vi "SubVI_Train_SVM.vi"(0 "Rest Epochs":dbl[][](array[numeric]), 1 "Repeat training?":bool=TRUE, 5 "Go Epochs in":dbl[][](array[numeric]), 9 "Max Passes":i32=15, 11 "error in (no error)":errorcluster, 12 "Gamma":dbl[](array[numeric])=[1.0, 5.0, 10.0, 50.0, 100.0, 0.2, 0.5, 0.8], 13 "C":dbl[](array[numeric])=[0.1, 1.0, 10.0, 100.0, 1000.0], 14 "Optimizer\nMetric":string="F1") -> (3 "Go Epochs out":dbl[][](array[numeric]), 4 "Hyperparameters":T1, 6 "Best (Metric)":dbl, 10 "Optimum Window Size":i32, 15 "error out":errorcluster)   [LabVIEW 2020]
uses:
  <vilib>/Analysis/Matrix/Numeric/Conversions/Matrix To Array - RM.vi
  Global 1.vi
  <vilib>/gmath/NI_Gmath.lvlib
  <vilib>/Analysis/Matrix/NI_Matrix.lvlib
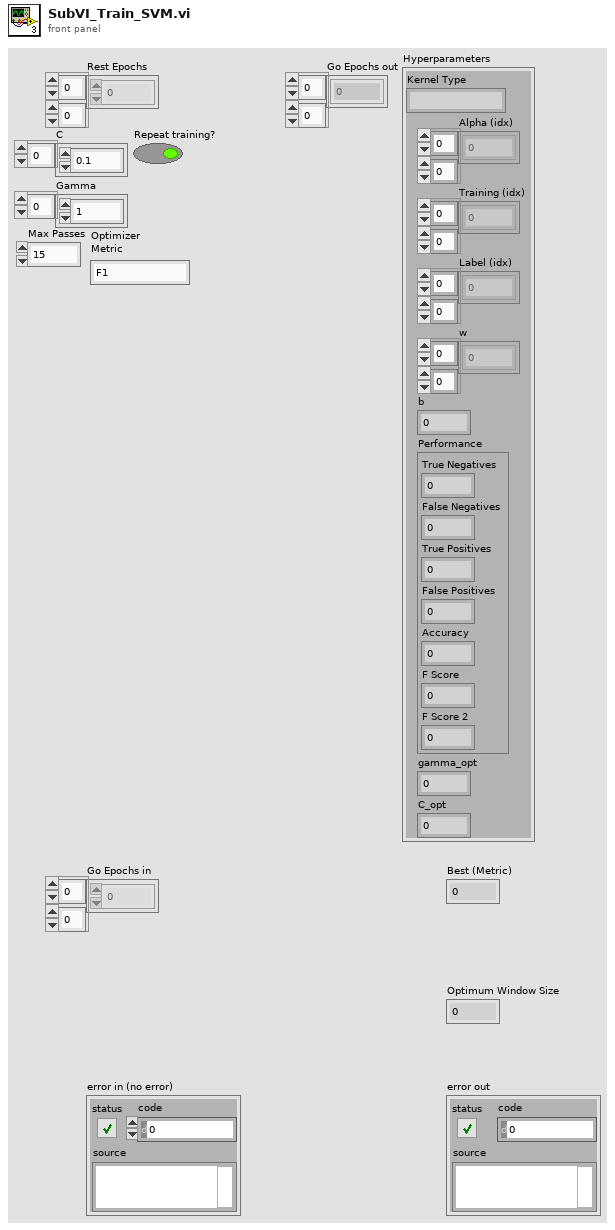
[diagram p1: front panel]
types:
  T1 = cluster{"Kernel Type":string, "Alpha (idx)":dbl[][], "Training (idx)":dbl[][], "Label (idx)":dbl[][], "w":dbl[][], "b":dbl, "Performance":cluster{"True Negatives":i32, "False Negatives":i32, "True Positives":i32, "False Positives":i32, "Accuracy":dbl, "F Score":dbl, "F Score 2":dbl}, "gamma_opt":dbl, "C_opt":dbl}
  T2 = typedef "NI_Matrix.lvlib/RealMatrix.ctl" = dbl[][]
  T3 = cluster{"True Negatives":i32, "False Negatives":i32, "True Positives":i32, "False Positives":i32, "Accuracy":dbl, "F1 Score":dbl, "Precision":dbl}
  T4 = cluster{"Kernel Type":string, "Alpha (idx)":dbl[][], "Training (idx)":dbl[][], "Label (idx)":dbl[][], "w":dbl[][], "b":dbl, "Performance":cluster{"True Negatives":i32, "False Negatives":i32, "True Positives":i32, "False Positives":i32, "Accuracy":dbl, "F1 Score":dbl, "Precision":dbl}, "gamma_opt":dbl, "C_opt":dbl}
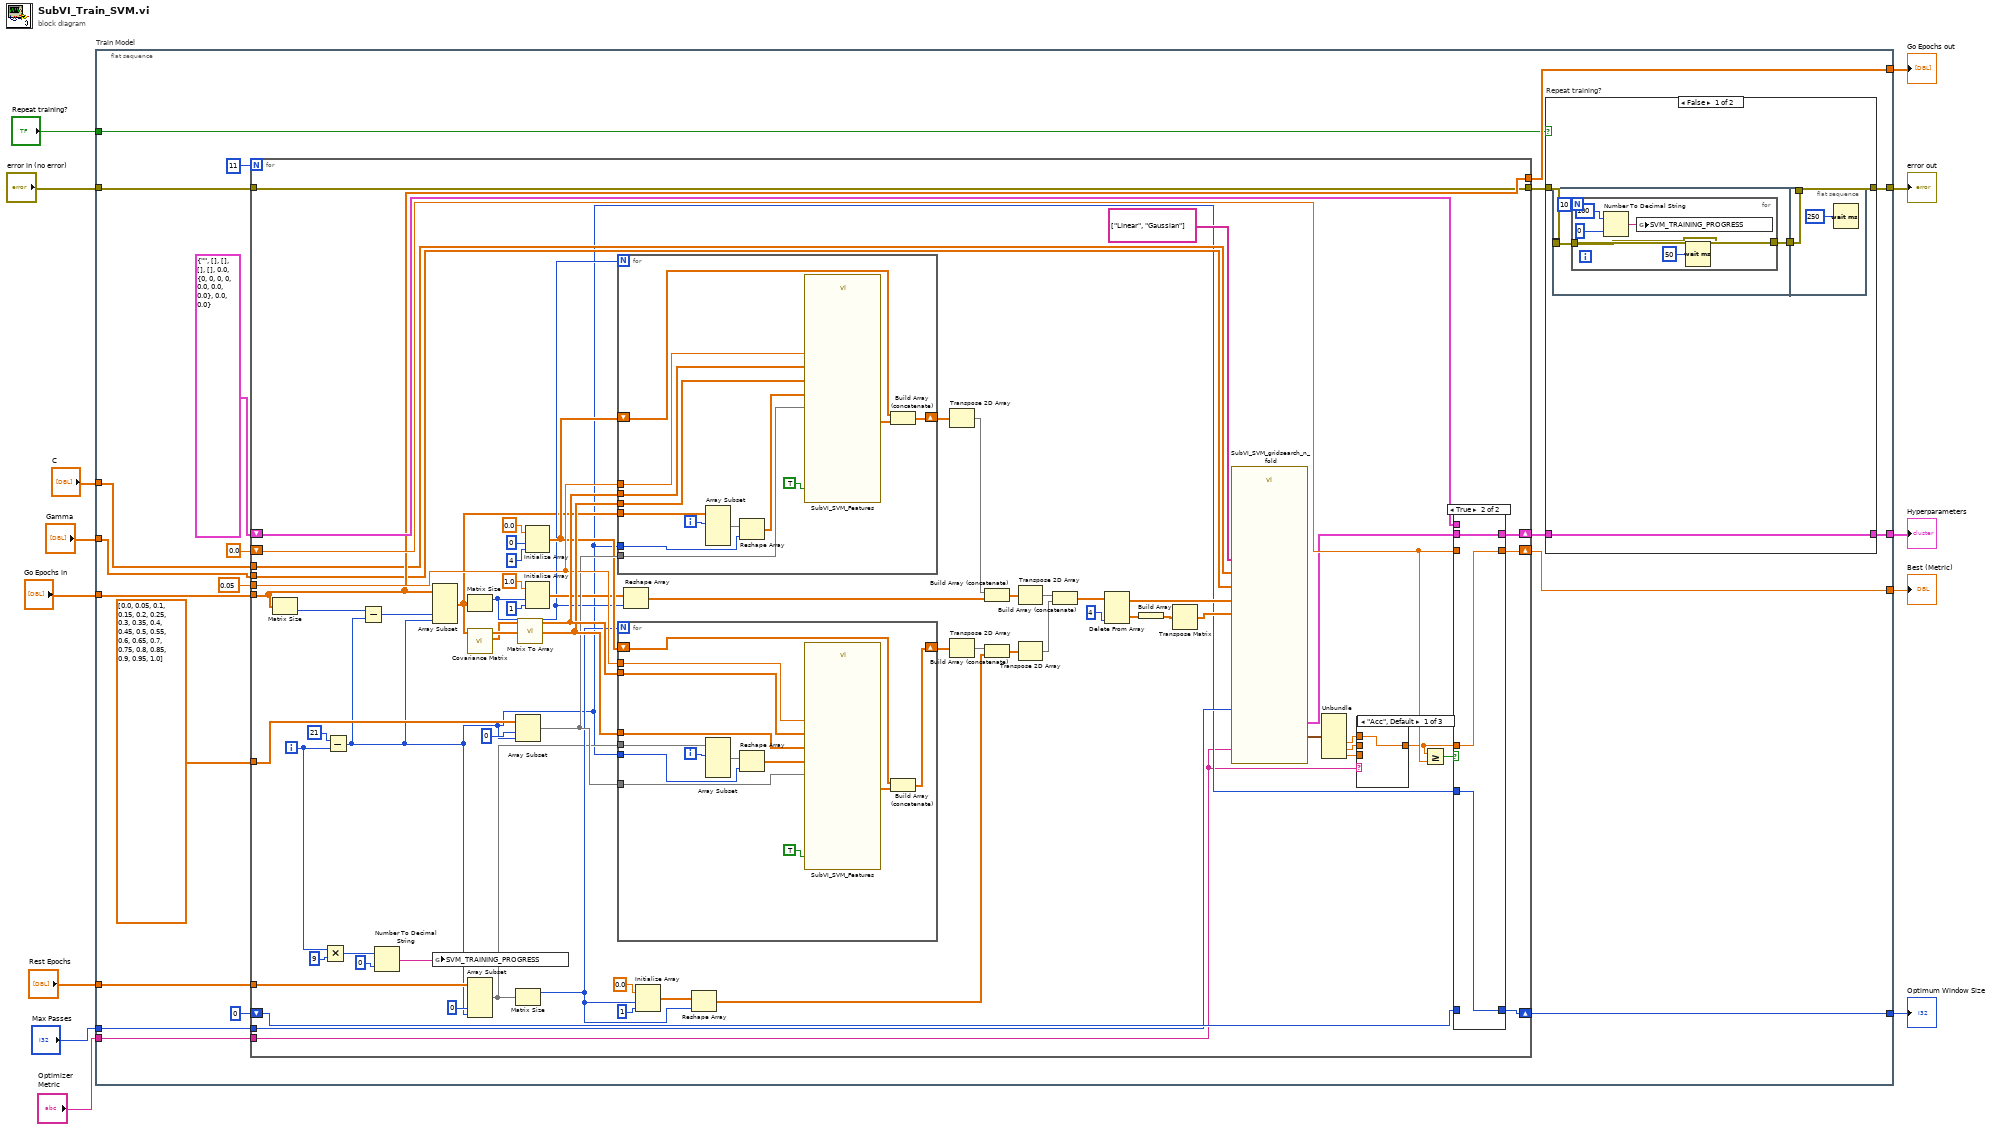
[diagram p0: block diagram]
diagram:
  n1 = flat-sequence "Train Model" {
    tunnel: "Go Epochs in" -> [w29]
    tunnel: "Rest Epochs" -> [w28]
    tunnel: [w27] -> w7
    tunnel: [w21] -> w2
    tunnel: [w26] -> w8
    tunnel: [w25] -> w9
    tunnel: [w15] -> w12
    tunnel: "error in (no error)" -> [w23]
    tunnel: "C" -> [w20]
    tunnel: "Gamma" -> [w19]
    tunnel: "Max Passes" -> [w18]
    tunnel: "Repeat training?" -> [w17]
    tunnel: "Optimizer\nMetric" -> [w14]
    frame #0 {
      n2 = for {
        N: 11 -> [_]
        tunnel: w29 -> [w71]
        tunnel: dbl[] [0.0, 0.05, 0.1, 0.15, 0.2, 0.25, 0.3, 0.35, 0.4, 0.45, 0.5, 0.55, 0.6, 0.65, 0.7, 0.75, 0.8, 0.85, 0.9, 0.95, 1.0] ("Sliding_window") -> [w117]
        tunnel: 0.05 ("dt") -> [w112]
        tunnel: w28 -> [w110]
        shift-right: [w75] -> w22
        shift-left: T1 {"Kernel Type"="", "Alpha (idx)"=[], "Training (idx)"=[], "Label (idx)"=[], "w"=[], "b"=0.0, "Performance"={"True Negatives"=0, "False Negatives"=0, "True Positives"=0, "False Positives"=0, "Accuracy"=0.0, "F Score"=0.0, "F Score 2"=0.0}, "gamma_opt"=0.0, "C_opt"=0.0} ("Hyperparameters") -> [w78]
        shift-right: [w73] -> w27
        shift-left: 0.0 -> [w74]
        shift-right: [w76] -> w25
        shift-left: 0 -> [w77]
        tunnel: [w71] -> w26
        tunnel: [w68] -> w16
        tunnel: w23 -> [w68]
        tunnel: w20 -> [w61]
        tunnel: w19 -> [w60]
        tunnel: w18 -> [w59]
        tunnel: w14 -> [w51]
        i -> [w63]
        n3 = Matrix Size(0:w71) -> (2:w69:i32)  [unwired: 1 out]
        n4 = Multiply(x=w63, y=9) -> (x*y=w64:i32)
        n5 = Subtract(x=21, y=w63) -> (x-y=w56:i32)
        n6 = Subtract(x=w69, y=w56) -> (x-y=w70:i32)
        n7 = Number To Decimal String(number=w64, width (-)=i16 0) -> (decimal integer string=w65:string)
        n8 = Array Subset(array=w71, index (col)=w70, length (col)=w56) -> (w87:dbl[][])  [unwired: 2 in]
        n9 = global write "Global 1.vi" "SVM_TRAINING_PROGRESS"(w65) -> ()
        n10 = Matrix Size(0:w87) -> (1:w90:i32)  [unwired: 1 out]
        n11 = call <vilib>:"Covariance Matrix.vi"("X"=w87) -> ("mean vector"=w114:dbl[], "covariance matrix V"=w118:T2)  [unwired: 9 in]
        n12 = Array Subset(array=w110, index (col)=0 ("index"), length (col)=w56) -> (w88:dbl[][])  [unwired: 2 in]
        n13 = Array Subset(array=w117, index=0, length=w56) -> (w109:dbl[])
        n14 = Matrix Size(0:w88) -> (1:w91:i32)  [unwired: 1 out]
        n15 = call-poly <vilib>:"Matrix To Array.vi"("Real Matrix"=w118) -> ("Real 2D Array"=w113:dbl[][])
        n16 = Initialize Array(0.0 ("element"), 0 ("dimension size"), 4 ("dimension size")) -> (w105:dbl[][])
        n17 = Initialize Array(1.0 ("element"), w90, 1 ("dimension size")) -> (w95:dbl[][])
        n18 = for {
          N: w90 -> [_]
          tunnel: w114 -> [w139]
          tunnel: w113 -> [w137]
          tunnel: w112 -> [w140]
          tunnel: w109 -> [w138]
          shift-right: [w135] -> w89
          shift-left: w105 -> [w136]
          tunnel: w87 -> [w133]
          tunnel: w56 -> [w131]
          i -> [w130]
          n19 = Array Subset(array=w133, index (row)=w130) -> (w132:dbl[][])  [unwired: 3 in]
          n20 = Reshape Array(w132, w131) -> (w129:dbl[])
          n21 = call "SubVI_SVM_Features.vi"("Sigma"=w137, "MU"=w139, "Scale?"=TRUE, "dt"=w140, "window_time"=w138, "Sliding_window"=w129) -> ("Features_array"=w134:dbl[])  [unwired: 1 in, 4 out]
          n22 = Build Array (concatenate)(w136, w134) -> (w135:dbl[][])
        }
        n23 = for {
          N: w91 -> [_]
          tunnel: w114 -> [w153]
          tunnel: w113 -> [w148]
          tunnel: w112 -> [w142]
          tunnel: w109 -> [w152]
          shift-right: [w149] -> w98
          shift-left: w105 -> [w151]
          tunnel: w88 -> [w147]
          tunnel: w56 -> [w143]
          i -> [w146]
          n24 = Array Subset(array=w147, index (row)=w146) -> (w145:dbl[][])  [unwired: 3 in]
          n25 = Reshape Array(w145, w143) -> (w144:dbl[])
          n26 = call "SubVI_SVM_Features.vi"("Sigma"=w148, "MU"=w153, "Scale?"=TRUE, "dt"=w142, "window_time"=w152, "Sliding_window"=w144) -> ("Features_array"=w150:dbl[])  [unwired: 1 in, 4 out]
          n27 = Build Array (concatenate)(w151, w150) -> (w149:dbl[][])
        }
        n28 = Reshape Array(w95, w90) -> (w94:dbl[])
        n29 = Initialize Array(0.0 ("element"), w91, 1 ("dimension size")) -> (w102:dbl[][])
        n30 = Reshape Array(w102, w91) -> (w101:dbl[])
        n31 = Transpose 2D Array(2D array=w89) -> (transposed array=w93:dbl[][])
        n32 = Transpose 2D Array(2D array=w98) -> (transposed array=w100:dbl[][])
        n33 = Build Array (concatenate)(w93, w94) -> (w92:dbl[][])
        n34 = Build Array (concatenate)(w100, w101) -> (w99:dbl[][])
        n35 = Transpose 2D Array(2D array=w92) -> (transposed array=w86:dbl[][])
        n36 = Transpose 2D Array(2D array=w99) -> (transposed array=w85:dbl[][])
        n37 = Build Array (concatenate)(w86, w85) -> (w84:dbl[][])
        n38 = Delete From Array(array=w84, index (col)=4 ("disabled index (col)")) -> (deleted portion=w82:dbl[], array with subset deleted=w80:dbl[][])  [unwired: 2 in]
        n39 = Build Array(w82) -> (w81:dbl[][])
        n40 = Transpose Matrix(1:w81) -> (0:w72:dbl[][])
        n41 = call "SubVI_SVM_gridsearch_n_fold.vi"("Max Passes"=w59, "Training Labels"=w72, "Training Data"=w80, "Array"=string[] ["Linear", "Gaussian"], "Optimizer\nMetric"=w51, "C"=w61, "Gamma"=w60) -> ("Performance"=w58:T3, "Hyperparameters"=w57:T4)  [unwired: 1 in, 6 out]
        n42 = Unbundle(w58) -> ("Accuracy"=w55:dbl, "F1 Score"=w54:dbl, "Precision"=w53:dbl)  [unwired: 4 out]
        n43 = case shown="\"Acc\", Default" w51 {
          tunnel: w53 -> [_ w120 _]
          tunnel: w54 -> [_ _ w121]
          tunnel: w55 -> [w119 _ _]
          tunnel: [w119 w120 w121] -> w52
          frame "Acc", Default {
          }
          frame "Prec" {
          }
          frame "F1" {
          }
        }
        n44 = Greater Or Equal?(x=w52, y=w74) -> (x >= y?=w79:bool)
        n45 = case shown="True" w79 {
          tunnel: w52 -> [_ w127]
          tunnel: [w124 w127] -> w73
          tunnel: w74 -> [w124 _]
          tunnel: [w123 w126] -> w76
          tunnel: w56 -> [_ w126]
          tunnel: w77 -> [w123 _]
          tunnel: w78 -> [w122 _]
          tunnel: [w122 w125] -> w75
          tunnel: w57 -> [_ w125]
          frame False {
          }
          frame True {
          }
        }
      }
      n46 = case "Repeat training?" shown="False" w17 {
        tunnel: w22 -> [w38 w50]
        tunnel: [w38 w50] -> w21
        tunnel: w16 -> [w37 w49]
        tunnel: [w36 w49] -> w15
        frame False {
          n47 = flat-sequence {
            tunnel: [w39] -> _
            tunnel: w37 -> [w40]
            tunnel: [w39] -> w35
            tunnel: [w47] -> w36
            tunnel: w35 -> [w47]
            frame #0 {
              n48 = for {
                N: 10 -> [_]
                tunnel: [w42] -> w39
                tunnel: w40 -> [w42]
                n49 = Number To Decimal String(number=100 ("y"), width (-)=i16 0) -> (decimal integer string=w46:string)
                n50 = global write "Global 1.vi" "SVM_TRAINING_PROGRESS"(w46) -> ()
                n51 = Wait (ms)(milliseconds to wait=u32 50) -> ()  [unwired: 1 out]
              }
            }
            frame #1 {
              n52 = Wait (ms)(milliseconds to wait=u32 250) -> ()  [unwired: 1 out]
            }
          }
        }
        frame True {
        }
      }
    }
  }
  "error out" <- w12
  "Optimum Window Size" <- w9
  "Go Epochs out" <- w8
  "Best (Metric)" <- w7
  "Hyperparameters" <- w2
